vi "Perform Self Test.vi"(8 "error in (no error)":errorcluster, 11 "Module ID":i32=-1) -> (0 "error out":errorcluster, 1 "timed out?":bool, 2 "Reply Payload":T1)   [LabVIEW 2015, in "Device Under Test_Cloneable_DQMH.lvlib"]
doc: "Request the Device Under Test to perform self test.\n_____\nCreated using Delacor QMH Event Scripter 1.0.0.50.\n____\nDelacor QMH Thermal Chamber Examples 4.0.0.21\nCopyright (c) 2018, Delacor"
uses:
  Device Under Test_Cloneable_DQMH.lvlib
  Perform Self Test (Reply Payload)--cluster.ctl
  Perform Self Test Argument--cluster.ctl
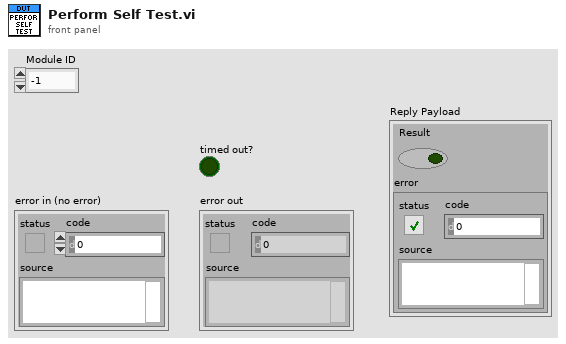
[diagram p1: front panel]
types:
  T1 = typedef "Device Under Test_Cloneable_DQMH.lvlib/Perform Self Test (Reply Payload)--cluster.ctl" = cluster{"Result":bool, "error":errorcluster}
  T2 = typedef "Device Under Test_Cloneable_DQMH.lvlib/Perform Self Test Argument--cluster.ctl" = cluster{"Module ID":i32, "Wait Notifier":refnum<notifier>}
  T3 = typedef "Device Under Test_Cloneable_DQMH.lvlib/Request Events--cluster.ctl" = cluster{"Stop Module":refnum<user-event>, "Show Panel":refnum<user-event>, "Hide Panel":refnum<user-event>, "Show Diagram":refnum<user-event>, "Set Power State":refnum<user-event>, "Perform Self Test":refnum<user-event>, "Update DUT Status":refnum<user-event>, "Get Module Execution Status":refnum<user-event>}
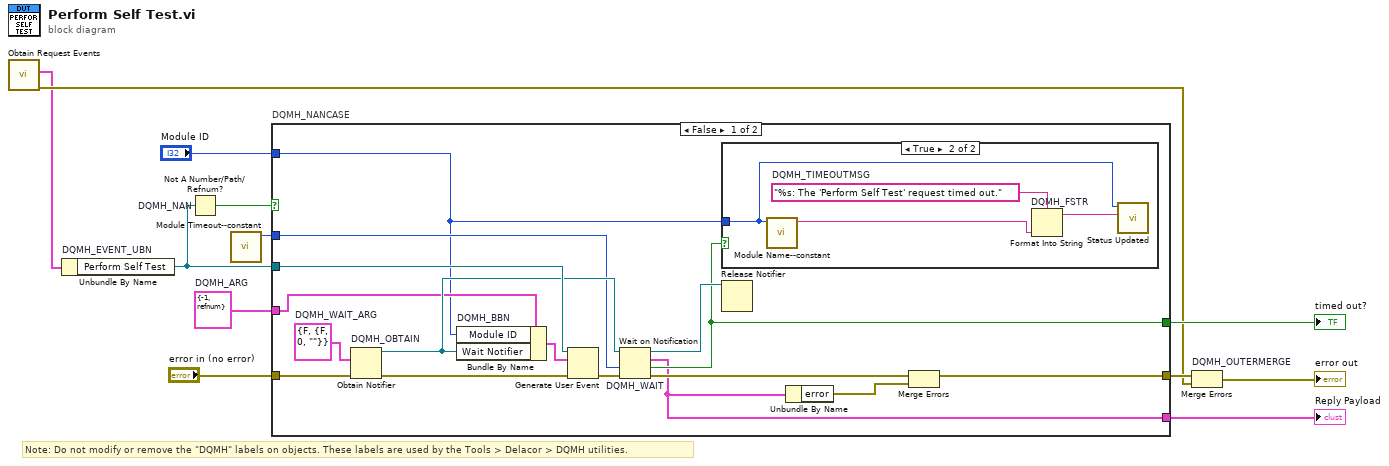
[diagram p0: block diagram]
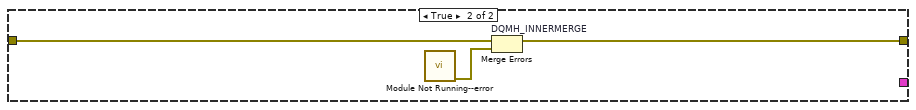
[diagram p3: hidden frame]
diagram:
  w6 = T2 {"Module ID"=-1, "Wait Notifier"=refnum}  # DQMH_ARG
  # "Note: Do not modify or remove the \"DQMH\" labels on objects. These labels are used by the Tools > Delacor > DQMH utilities."
  n1 = call "Obtain Request Events.vi"() -> ("error out"=w4:errorcluster, "Device Under Test_Cloneable_DQMH Request Events"=w3:T3)  [unwired: 10 in]
  n2 = Unbundle By Name "DQMH_EVENT_UBN"(w3) -> ("Perform Self Test"=w9:refnum<user-event>)
  n3 = Not A Number/Path/Refnum? "DQMH_NAN"(number/path/refnum=w9) -> (NaN/Path/Refnum?=w8:bool)
  n4 = call "Module Timeout--constant.vi"() -> ("Module Timeout"=w5:i32)  [unwired: 11 in]
  n5 = case "DQMH_NANCASE" shown="False" w8 {
    tunnel: "error in (no error)" -> [w28 w35]
    tunnel: w9 -> [w26 _]
    tunnel: [w17 w34] -> w10
    tunnel: [w19 _] -> w7
    tunnel: w6 -> [w14 _]
    tunnel: w5 -> [w18 _]
    tunnel: [w16 _] -> w2
    tunnel: "Module ID" -> [w13 _]
    frame False {
      w23 = T1 {"Result"=FALSE, "error"={"status"=FALSE, "code"=0, "source"=""}}  # DQMH_WAIT_ARG
      n6 = Obtain Notifier "DQMH_OBTAIN"(notification data type=w23, error in (no error)=w28) -> (notifier out=w21:refnum<notifier>, error out=w24:errorcluster)  [unwired: 2 in, 1 out]
      n7 = Bundle By Name "DQMH_BBN"(cluster=w14, "Module ID"=w13, "Wait Notifier"=w21) -> (w25:T2)
      n8 = Generate User Event(user event=w26, event data cluster=w25, error in=w24) -> (error out=w27:errorcluster)  [unwired: 1 in, 1 out]
      n9 = Wait on Notification "DQMH_WAIT"(notifier=w21, timeout in ms (-1)=w18, error in (no error)=w27) -> (notifier out=w20:refnum<notifier>, notification=w16:T1, timed out?=w19:bool, error out=w22:errorcluster)  [unwired: 1 in]
      n10 = case shown="True" w19 {
        tunnel: w13 -> [_ w29]
        frame False {
        }
        frame True {
          w32 = "%s: The 'Perform Self Test' request timed out."  # DQMH_TIMEOUTMSG
          n11 = call "Module Name--constant.vi"("Module ID"=w29) -> ("Module Name"=w31:string)  [unwired: 10 in]
          n12 = Format Into String "DQMH_FSTR"(format string=w32, w31) -> (resulting string=w30:string)  [unwired: 2 in, 1 out]
          n13 = call "Status Updated.vi"("Status"=w30, "Module ID"=w29) -> ()  [unwired: 9 in, 1 out]
        }
      }
      n14 = Release Notifier(notifier=w20) -> ()  [unwired: 2 in, 3 out]
      n15 = Unbundle By Name(w16) -> ("error"=w15:errorcluster)
      n16 = Merge Errors(w22, w15) -> (w17:errorcluster)
    }
    frame True {
      n17 = call "Module Not Running--error.vi"() -> ("error out"=w33:errorcluster)  [unwired: 11 in]
      n18 = Merge Errors "DQMH_INNERMERGE"(w35, w33) -> (w34:errorcluster)
    }
  }
  "timed out?" <- w7
  "Reply Payload" <- w2
  n19 = Merge Errors "DQMH_OUTERMERGE"(w10, w4) -> (→"error out":errorcluster)
